vi "ifr2025 Set FSK Ext.vi"(8 "error in (no error)":errorcluster {"code" format="%.0x"}, 9 "FM1 State (Off)":bool, 10 "FM1 Deviation (0.0)":dbl, 11 "instrument handle":refnum<visa-resource-name>) -> (0 "error out":errorcluster {"code" format="%.0x"}, 3 "instrument handle out":refnum<visa-resource-name>)   [LabVIEW 2009]
doc: "This function controls FM1 for FSK mode by setting channel 1 of the modulation oscillator."
uses:
  Ifr2025_32.dll
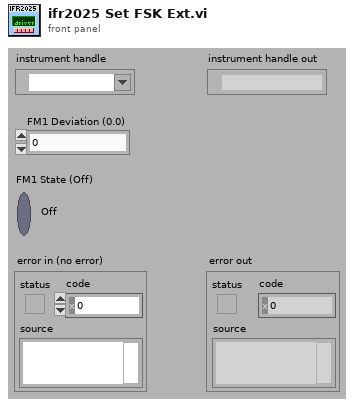
[diagram p1: front panel]
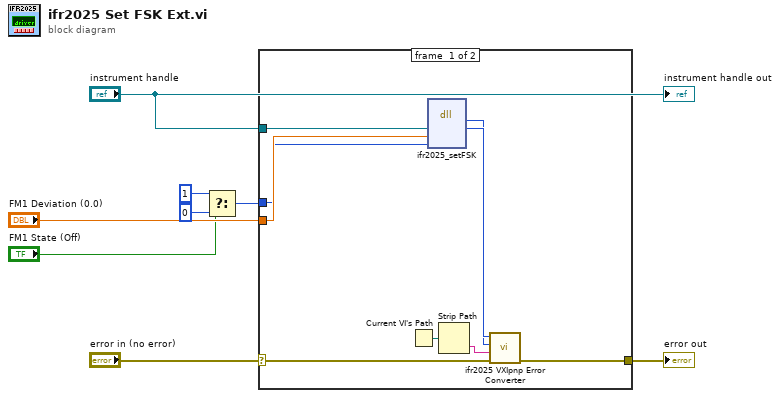
[diagram p0: block diagram]
diagram:
  n1 = Select(t=u16 1, s="FM1 State (Off)", f=u16 0) -> (s? t:f=w1:u16)
  n2 = case shown="No Error" "error in (no error)" {
    selector: "error in (no error)" -> [w12 w18]
    tunnel: [w11 w18] -> w8
    tunnel: "instrument handle" -> [w16 _]
    tunnel: "FM1 Deviation (0.0)" -> [w10 _]
    tunnel: w1 -> [w9 _]
    frame #0 {
      n3 = Current VI's Path() -> (path=w17:path)
      n4 = dll-call lib="P:/inst/Marconi 2024 Signal Generator/source/labview/ifr2025/ifr2025/ifr2025_*.*" fn="ifr2025_setFSK"("vi"=w16, "FM1 Deviation"=w10, "FM1 State"=w9) -> (w14:i32, "vi"=w15:u32)  [unwired: 5 in, 2 out]
      n5 = Strip Path(path=w17) -> (name=w13:string)  [unwired: 1 out]
      n6 = call "ifr2025 VXIpnp Error Converter.vi"("error in (no error)"=w12, "name of VI (\"\")"=w13, "CVI error code (0)"=w14, "instrument handle"=w15) -> ("error out"=w11:errorcluster)  [unwired: 7 out]
    }
    frame #1 {
    }
  }
  "error out" <- w8
  "instrument handle out" <- "instrument handle"
